vi "1TableGenerateData.vi"(7 "HeaderPrefix":string, 8 "error in (no error)":errorcluster, 11 "Cluster Variant":variant) -> (0 "error out":errorcluster, 1 "Data":string[](array[string]), 2 "Headers":string[](array[string]), 3 "Table Name":string, 5 "LV Data Types":T1[](array[typedef]) format="%.0x")   [LabVIEW 2014, in "TableLogger_Actor.lvlib" / "TableLogger_Actor.lvclass"]
uses:
  TableLogger_Actor.lvclass
  <userlib>/_OpenG.lib/lvdata/lvdata.llb/Type Descriptor Enumeration__ogtk.ctl
panel:
  # "Connector Pane"
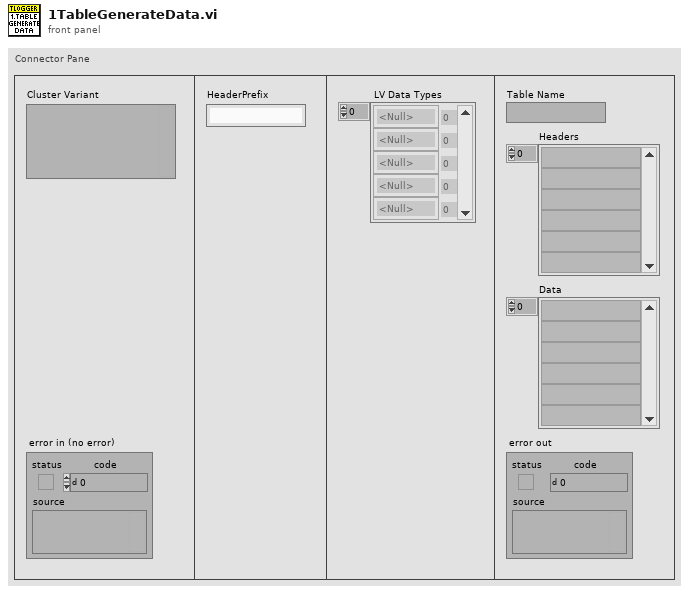
[diagram p1: front panel]
types:
  T1 = typedef "Type Descriptor Enumeration__ogtk.ctl" = enum8{"<Null>", "I8", "I16", "I32", "I64", "U8", "U16", "U32", "U64", "SGL", "DBL", "EXT", "CSG", "CDB", "CXT", "0x0F", "0x10", "0x11", "0x12", "0x13", "0x14", "Enum U8", "Enum U16", "Enum U32", "Enum U64", "SGL PQ", "DBL PQ", "EXT PQ", "CSG PQ", "CDB PQ", "CXT PQ", "0x1F", "0x20", "Boolean", "0x22", "0x23", "0x24", "0x25", "0x26", "0x27", "0x28", "0x29", "0x2A", "0x2B", "0x2C", "0x2D", "0x2E", "0x2F", "String", "0x31", "Path", "Pict", "0x34", "0x35", "0x36", "DAQ", "0x38", "0x39", "0x3A", "0x3B", "0x3C", "0x3D", "0x3E", "0x3F", "Array", "0x41", "0x42", "0x43", "0x44", "0x45", "0x46", "0x47", "0x48", "0x49", "0x4A", "0x4B", "0x4C", "0x4D", "0x4E", "0x4F", "Cluster", "0x51", "0x52", "Variant", "Waveform", "0x55", "0x56", "0x57", "0x58", "0x59", "0x5A", "0x5B", "0x5C", "0x5D", "0x5E", "0x5F", "0x60", "0x61", "0x62", "0x63", "0x64", "0x65", "0x66", "0x67", "0x68", "0x69", "0x6A", "0x6B", "0x6C", "0x6D", "0x6E", "0x6F", "Refnum"}
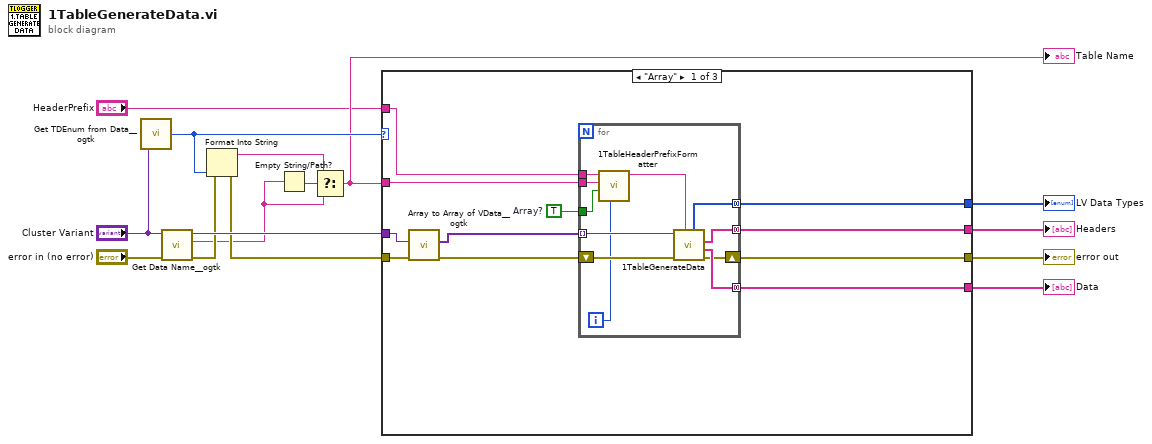
[diagram p0: block diagram]
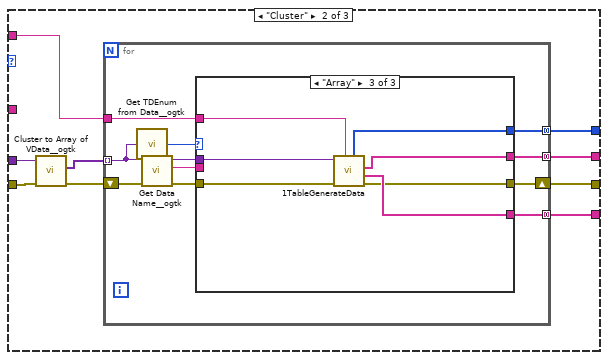
[diagram p2: hidden frame]
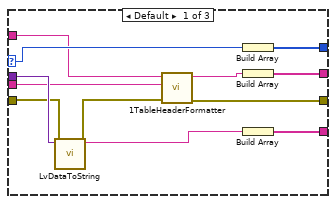
[diagram p3: hidden frame]
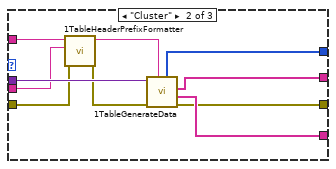
[diagram p4: hidden frame]
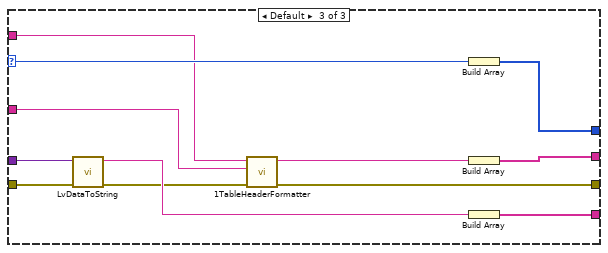
[diagram p5: hidden frame]
diagram:
  n1 = call <userlib>:"Get TDEnum from Data__ogtk.vi"("Data"="Cluster Variant") -> ("Type Descriptor Enumeration"=w7:T1)  [unwired: 4 in]
  n2 = call <userlib>:"Get Data Name__ogtk.vi"("error in (no error)"="error in (no error)", "Data"="Cluster Variant") -> ("error out"=w5:errorcluster, "Data Name"=w3:string, "Data dup"=w9:variant)  [unwired: 7 in]
  n3 = Format Into String(error in=w5, w7) -> (resulting string=w6:string, error out=w4:errorcluster)  [unwired: 2 in]
  n4 = Empty String/Path?(string/path=w3) -> (empty?=w8:bool)
  n5 = Select(t=w6, s=w8, f=w3) -> (s? t:f=w2:string)
  "Table Name" <- w2
  n6 = case shown="\"Array\"" w7 {
    selector: w7 -> [_ _ w95]
    tunnel: w9 -> [w20 w44 w93]
    tunnel: [w26 w46 w97] -> w15
    tunnel: [w25 w45 w98] -> w14
    tunnel: w4 -> [w21 w39 w94]
    tunnel: [w24 w41 w90] -> w13
    tunnel: [w23 w40 w96] -> w12
    tunnel: "HeaderPrefix" -> [w19 w38 w89]
    tunnel: w2 -> [w18 _ w88]
    frame "Array" {
      w16 = TRUE  # Array?
      n7 = call <userlib>:"Array to Array of VData__ogtk.vi"("error in (no error)"=w21, "MultiD Array"=w20) -> ("error out"=w17:errorcluster, "1D Array of Variants"=w22:variant[])  [unwired: 8 in]
      n8 = for {
        tunnel: [w37] -> w26 mode=concatenating
        tunnel: [w36] -> w25 mode=concatenating
        tunnel: [w34] -> w23 mode=concatenating
        tunnel: w22 -> [w33] mode=indexing
        tunnel: w19 -> [w31]
        shift-right: [w35] -> w24
        shift-left: w17 -> [w32]
        tunnel: w18 -> [w29]
        tunnel: w16 -> [w28]
        i -> [w27]
        n9 = call "1TableHeaderPrefixFormatter.vi"("ArrayIndex"=w27, "Array?"=w28, "Added HeaderPrefix"=w29, "Existing HeaderPrefix"=w31) -> ("HeaderPrefix"=w30:string)  [unwired: 6 in, 1 out]
        n10 = call "1TableGenerateData.vi"("HeaderPrefix"=w30, "error in (no error)"=w32, "Cluster Variant"=w33) -> ("error out"=w35:errorcluster, "Data"=w36:string[], "Headers"=w37:string[], "LV Data Types"=w34:T1[])  [unwired: 4 in, 1 out]
      }
    }
    frame "Cluster" {
      n11 = call <userlib>:"Cluster to Array of VData__ogtk.vi"("error in (no error)"=w39, "Cluster"=w44) -> ("error out"=w42:errorcluster, "Array of VData"=w43:variant[])  [unwired: 8 in]
      n12 = for {
        tunnel: w43 -> [w50] mode=indexing
        tunnel: [w57] -> w46 mode=concatenating
        tunnel: [w56] -> w45 mode=concatenating
        shift-right: [w55] -> w41
        shift-left: w42 -> [w52]
        tunnel: [w53] -> w40 mode=concatenating
        tunnel: w38 -> [w47]
        n13 = call <userlib>:"Get TDEnum from Data__ogtk.vi"("Data"=w50) -> ("Type Descriptor Enumeration"=w54:T1)  [unwired: 4 in]
        n14 = call <userlib>:"Get Data Name__ogtk.vi"("error in (no error)"=w52, "Data"=w50) -> ("error out"=w51:errorcluster, "Data Name"=w48:string, "Data dup"=w49:variant)  [unwired: 7 in]
        n15 = case shown="\"Array\"" w54 {
          selector: w54 -> [w67 _ _]
          tunnel: w49 -> [w63 w78 w85]
          tunnel: [w69 w79 w86] -> w57
          tunnel: [w66 w77 w84] -> w56
          tunnel: w51 -> [w62 w71 w80]
          tunnel: [w64 w76 w83] -> w55
          tunnel: [w68 w75 w82] -> w53
          tunnel: w48 -> [w58 w73 _]
          tunnel: w47 -> [w59 w74 w81]
          frame Default {
            n16 = call "LvDataToString.vi"("error in (no error)"=w62, "Variant"=w63) -> ("error out"=w60:errorcluster, "String Value"=w61:string)  [unwired: 8 in]
            n17 = call "1TableHeaderFormatter.vi"("error in (no error)"=w60, "Data Name"=w58, "HeaderPrefix"=w59) -> ("error out"=w64:errorcluster, "HeaderOut"=w65:string)  [unwired: 7 in]
            n18 = Build Array(w67) -> (w68:T1[])
            n19 = Build Array(w65) -> (w69:string[])
            n20 = Build Array(w61) -> (w66:string[])
          }
          frame "Cluster" {
            n21 = call "1TableHeaderPrefixFormatter.vi"("error in"=w71, "Added HeaderPrefix"=w73, "Existing HeaderPrefix"=w74) -> ("error out"=w70:errorcluster, "HeaderPrefix"=w72:string)  [unwired: 7 in]
            n22 = call "1TableGenerateData.vi"("HeaderPrefix"=w72, "error in (no error)"=w70, "Cluster Variant"=w78) -> ("error out"=w76:errorcluster, "Data"=w77:string[], "Headers"=w79:string[], "LV Data Types"=w75:T1[])  [unwired: 4 in, 1 out]
          }
          frame "Array" {
            n23 = call "1TableGenerateData.vi"("HeaderPrefix"=w81, "error in (no error)"=w80, "Cluster Variant"=w85) -> ("error out"=w83:errorcluster, "Data"=w84:string[], "Headers"=w86:string[], "LV Data Types"=w82:T1[])  [unwired: 4 in, 1 out]
          }
        }
      }
    }
    frame Default {
      n24 = call "LvDataToString.vi"("error in (no error)"=w94, "Variant"=w93) -> ("error out"=w91:errorcluster, "String Value"=w92:string)  [unwired: 8 in]
      n25 = call "1TableHeaderFormatter.vi"("error in (no error)"=w91, "Data Name"=w88, "HeaderPrefix"=w89) -> ("error out"=w90:errorcluster, "HeaderOut"=w87:string)  [unwired: 7 in]
      n26 = Build Array(w95) -> (w96:T1[])
      n27 = Build Array(w87) -> (w97:string[])
      n28 = Build Array(w92) -> (w98:string[])
    }
  }
  "Headers" <- w15
  "Data" <- w14
  "error out" <- w13
  "LV Data Types" <- w12
